vi "Set TD Header Subset.vi"(8 "错误输入":errorcluster, 10 "Type Descriptor Head Subse":u16[](array[numeric]), 11 "Data Name":string) -> (0 "错误输出":errorcluster, 3 "Type Descriptor Head Subset输出":u16[](array[numeric]))   [LabVIEW 2012, in "TD Tools.lvlib"]
uses:
  TD Tools.lvlib
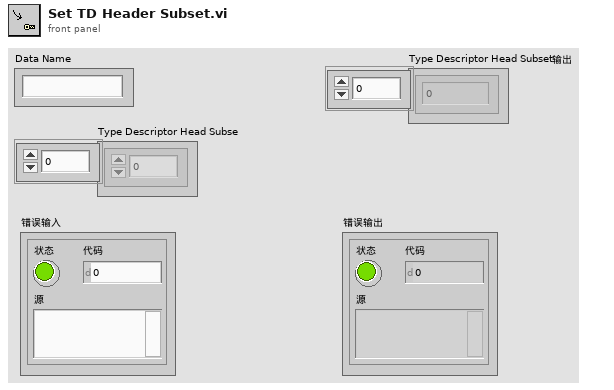
[diagram p1: front panel]
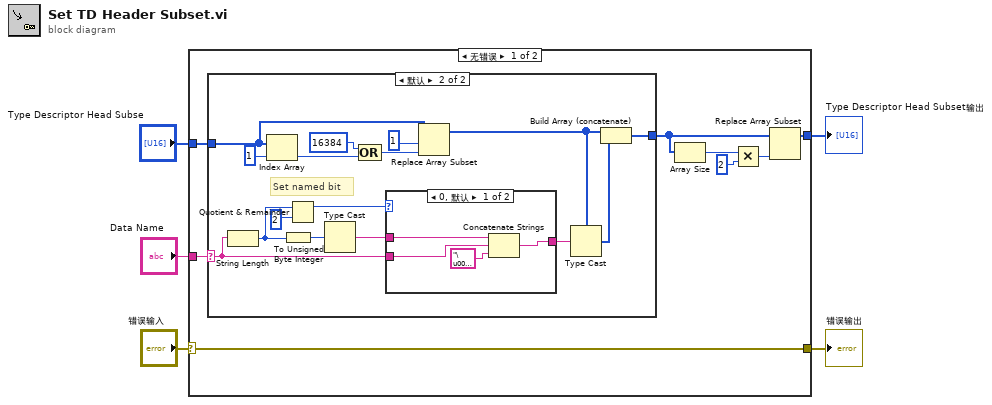
[diagram p0: block diagram]
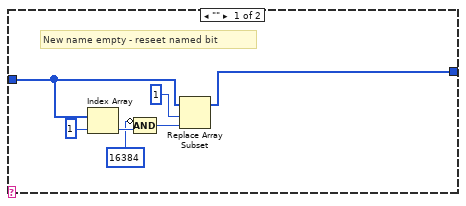
[diagram p2: hidden frame]
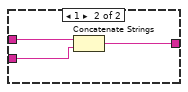
[diagram p3: hidden frame]
diagram:
  n1 = case shown="无错误" "错误输入" {
    selector: "错误输入" -> [w6 w45]
    tunnel: "Data Name" -> [w13 _]
    tunnel: [w12 w44] -> w4
    tunnel: "Type Descriptor Head Subse" -> [w7 w44]
    tunnel: [w6 w45] -> w1
    frame No Error {
      n2 = case shown="默认" w13 {
        selector: w13 -> [_ w28]
        tunnel: w7 -> [w20 w36]
        tunnel: [w15 w25] -> w11
        frame "" {
          # "New name empty - reseet named bit"
          n3 = Index Array(array=w20, index=1 ("Index")) -> (element=w18:u16)
          n4 = Compound Arithmetic op=AND(invert i16 16384 ("Input"), w18) -> (w17:u16)
          n5 = Replace Array Subset(array=w20, new element=w17, index=1 ("Index")) -> (w15:u16[])
        }
        frame Default {
          # "Set named bit"
          n6 = String Length(string=w28) -> (length=w24:i32)
          n7 = Index Array(array=w36, index=1 ("Index")) -> (element=w32:u16)
          n8 = To Unsigned Byte Integer(number=w24) -> (unsigned 8bit integer=w23:u8)
          n9 = Quotient & Remainder(x=w24, y=2) -> (x-y*floor(x/y)=w30:i32)  [unwired: 1 out]
          n10 = Type Cast(x=w23) -> (*(type *) &x=w22:string)  [unwired: 1 in]
          n11 = Compound Arithmetic op=OR(i16 16384 ("Input"), w32) -> (w34:u16)
          n12 = case shown="0, 默认" w30 {
            tunnel: [w40 w41] -> w29
            tunnel: w28 -> [w39 w42]
            tunnel: w22 -> [w37 w43]
            frame 0, Default {
              n13 = Concatenate Strings(w37, w39, "\u0000" ("Substring")) -> (w40:string)
            }
            frame 1 {
              n14 = Concatenate Strings(w43, w42) -> (w41:string)
            }
          }
          n15 = Replace Array Subset(array=w36, new element=w34, index=1 ("Index")) -> (w26:u16[])
          n16 = Type Cast(type=w26, x=w29) -> (*(type *) &x=w27:u16[])
          n17 = Build Array (concatenate)(w26, w27) -> (w25:u16[])
        }
      }
      n18 = Array Size(array=w11) -> (size(s)=w8:i32)
      n19 = Multiply(x=w8, y=2) -> (x*y=w10:i32)
      n20 = Replace Array Subset(array=w11, new element=w10) -> (w12:u16[])  [unwired: 1 in]
    }
    frame Error {
    }
  }
  "Type Descriptor Head Subset输出" <- w4
  "错误输出" <- w1
